vi "Decodejpg.vi"(8 "error in (no error)":errorcluster, 10 "name":string, 11 "Refnum in":T1) -> (0 "error out":errorcluster, 3 "Refnum out":T1(plugin-control))   [LabVIEW 2017]
uses:
  <vilib>/vision/Image Controls.llb/IMAQ Image.ctl
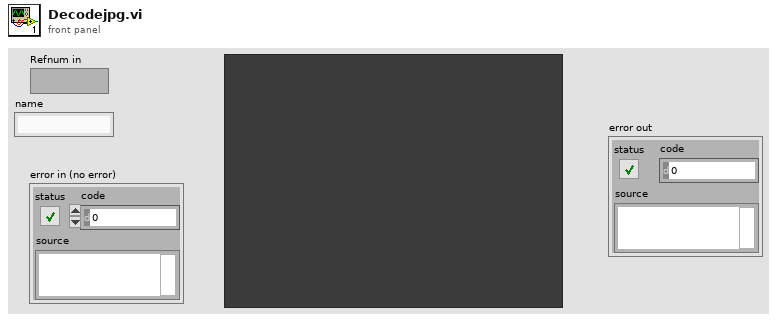
[diagram p1: front panel]
types:
  T1 = typedef "IMAQ Image.ctl" = refnum<image>
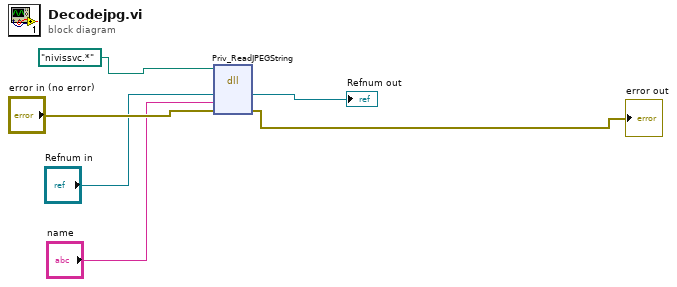
[diagram p0: block diagram]
diagram:
  n1 = dll-call lib="nivissvc.*" fn="Priv_ReadJPEGString"(path in=path "nivissvc.*", "image"="Refnum in", "name"="name", "err"="error in (no error)") -> ("image"=→"Refnum out":T1, "err"=→"error out":errorcluster)  [unwired: 3 in, 3 out]
